vi "Teleop.vi"(10 "Match Info":T1={"Autonomous Elapsed Seconds"=0.0, "TeleOp Elapsed Seconds"=0.0, "Disabled Elapsed Seconds"=0.0, "Visited Autonomous"=FALSE, "Visited TeleOp"=FALSE, "Visited Disabled"=FALSE, "Autonomous Settings"={"Autonomous Style"=enum."Independent", "VI Refnum"=refnum}}, 11 "Call Context":T2) -> ()   [LabVIEW 2012]
doc: "This VI is called for each TeleOp packet received from the DS where the robot is not disabled. It is often used to read from the joysticks and update I/O or to update setpoints for timed control loops. It should complete and return within 20 milliseconds or it may miss DS packets."
uses:
  <vilib>/Rock Robotics/WPI/DriverStation/WPI_DriverStationDerivedRobotMode.ctl
  <vilib>/Rock Robotics/WPI/DriverStation/WPI_DriverStationMatch Info.ctl
  <vilib>/Rock Robotics/WPI/Relay/WPI_RelayValue.ctl
  Robot Global Data.vi
  <vilib>/Rock Robotics/WPI/Joystick/WPI_JoystickGetSetRefNum.vi
  <vilib>/Rock Robotics/WPI/RobotDrive/WPI_RobotDriveGetSetRefNum.vi
panel:
  out "Numeric 1":dbl(slide) scale=0.0..100.0
  out "Boolean 2":bool
  out "Boolean 1":bool
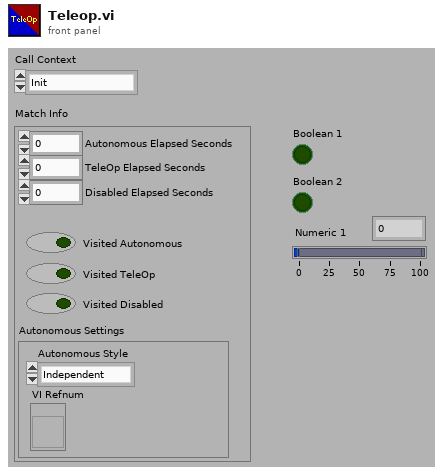
[diagram p1: front panel]
types:
  T1 = typedef "WPI_DriverStationMatch Info.ctl" = cluster{"Autonomous Elapsed Seconds":dbl, "TeleOp Elapsed Seconds":dbl, "Disabled Elapsed Seconds":dbl, "Visited Autonomous":bool, "Visited TeleOp":bool, "Visited Disabled":bool, "Autonomous Settings":cluster{"Autonomous Style":enum16{"Iterative", "Independent"}, "VI Refnum":refnum<vi>}}
  T2 = typedef "WPI_DriverStationDerivedRobotMode.ctl" = enum16{"Init", "Execute", "Stop"}
  T3 = typedef "WPI_JoystickDevRef.ctl" = cluster{"Device":T4}
  T4 = typedef "WPI_JoystickDeviceEnum.ctl" = enum16{"USB 1", "USB 2", "USB 3", "USB 4", "Kinect 1", "Kinect 2"}
  T5 = typedef "WPI_JoystickButtonState.ctl" = cluster{"Button 1":bool, "Button 2":bool, "Button 3":bool, "Button 4":bool, "Button 5":bool, "Button 6":bool, "Button 7":bool, "Button 8":bool, "Button 9":bool, "Button 10":bool, "Button 11":bool, "Button 12":bool}
  T6 = typedef "WPI_RelayValue.ctl" = enum16{"Off", "On", "Forward", "Reverse"}
  T7 = cluster{"axis 1 (x)":dbl, "axis 2 (y)":dbl, "axis 3 (throttle)":dbl, "axis 4":dbl, "axis 5":dbl, "axis 6":dbl}
  T8 = typedef "WPI_RelayDevRef.ctl" = cluster{"DevStatus":errorcluster, "Relay Channel":T9, "Digital Module":T10, "Relay Direction":T11}
  T9 = typedef "FPGA_DIORelayChannel.ctl" = enum8{"Relay 1", "Relay 2", "Relay 3", "Relay 4", "Relay 5", "Relay 6", "Relay 7", "Relay 8", "Invalid"}
  T10 = typedef "FPGA_TypedefDigitalModule.ctl" = enum16{"Digital Module 1", "Digital Module 2"}
  T11 = typedef "WPI_RelayDirection.ctl" = enum16{"Both directions", "Forward only", "Reverse only"}
  T12 = typedef "WPI_MotorControlDeviceRef.ctl" = cluster{"DeviceStatus":errorcluster, "Type":enum16{"PWM", "CAN"}, "PWM":cluster{"Digital Module":T10, "PWM Channel":T13, "DeadBand":T14}, "CAN":cluster{"Device Number":u8, "Control Mode":T15, "Semaphore":T16, "Max Vout":dbl}, "Invert":bool, "TransformRef":T17, "InvTransformRef":T17}
  T13 = typedef "FPGA_DIOPWMChannel.ctl" = enum8{"PWM 1", "PWM 2", "PWM 3", "PWM 4", "PWM 5", "PWM 6", "PWM 7", "PWM 8", "PWM 9", "PWM 10", "Invalid"}
  T14 = typedef "WPI_PWMDeadband.ctl" = cluster{"Name":string, "maxPositivePwm":i32, "minPositivePwm":i32, "centerPwm":i32, "maxNegativePwm":i32, "minNegativePwm":i32, "angularRange":u16}
  T15 = typedef "WPI_CANJaguar_ControlMode.ctl" = enum8{"Percent VBus", "Current", "Speed", "Position", "Voltage"}
  T16 = typedef "Semaphore RefNum" = refnum<k1>
  T17 = typedef "WPI_PWMTransform_ConPane.ctl" = refnum<vi>
  T18 = typedef "WPI_RobotDriveDevRef.ctl" = cluster{"DevStatus":errorcluster, "Motors[]":T12[], "Square Inputs":bool, "Max Output":dbl, "Isochronous":bool}
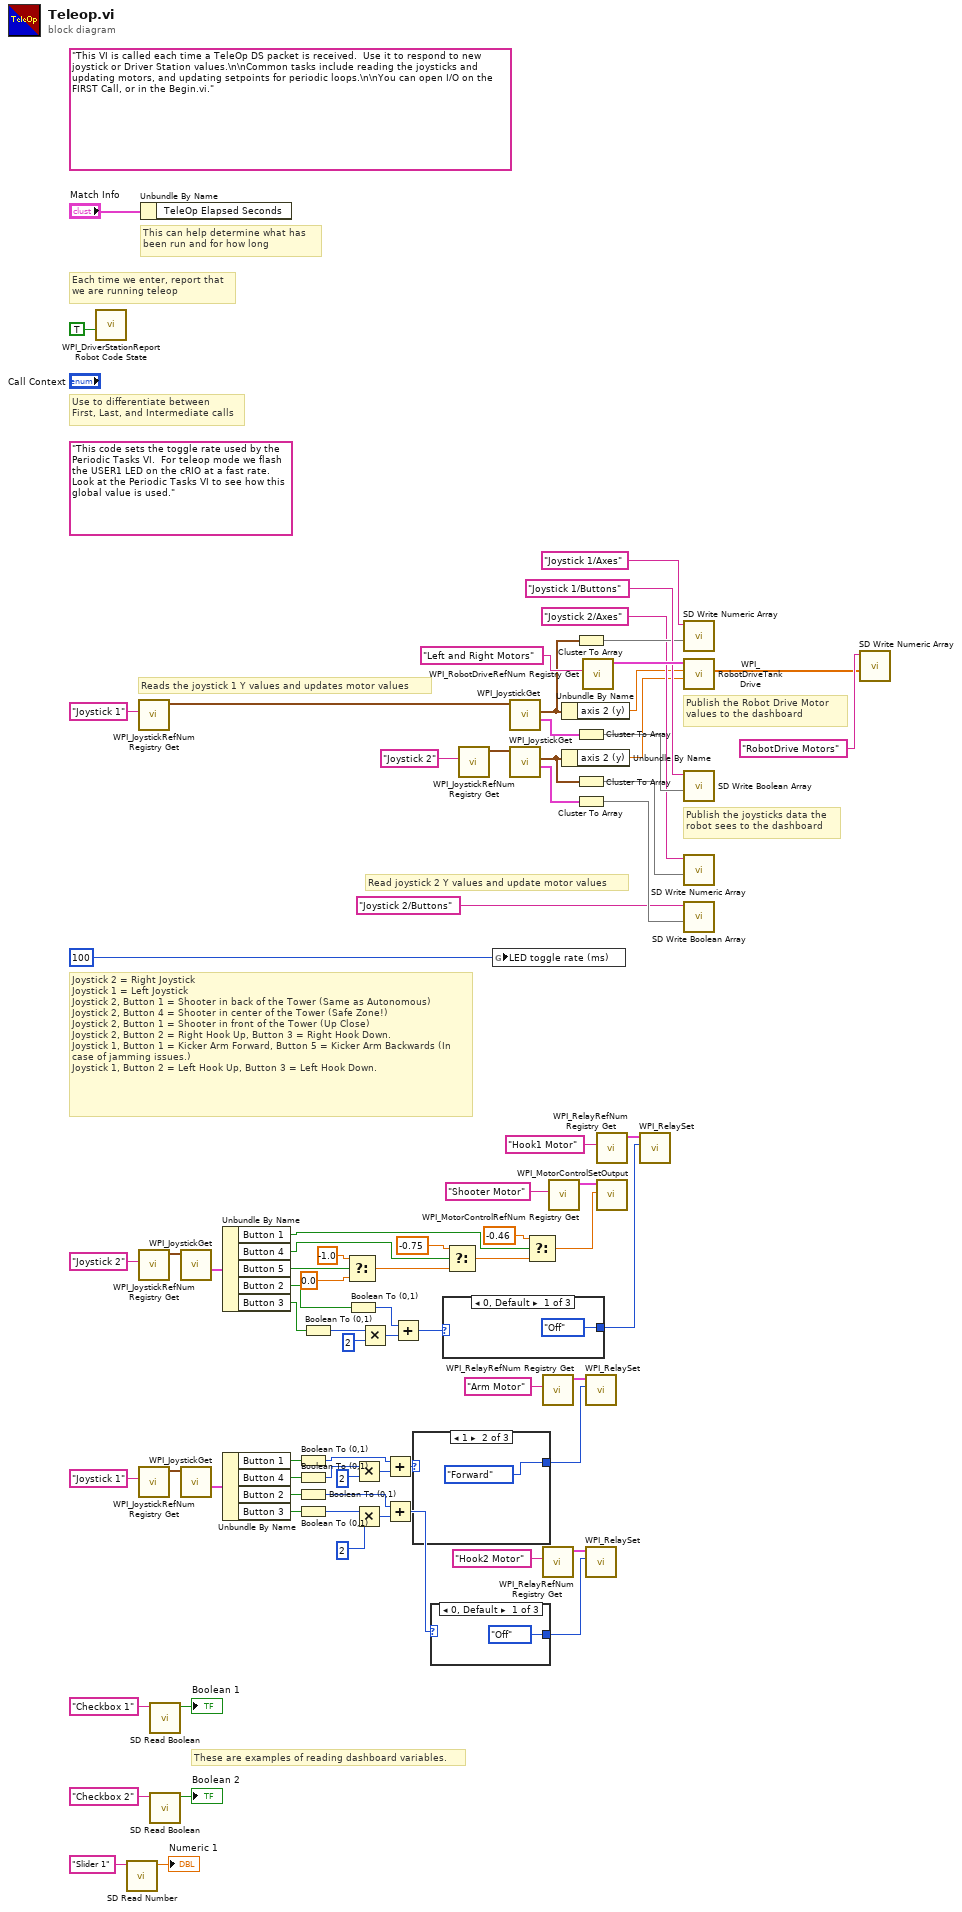
[diagram p0: block diagram]
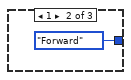
[diagram p2: hidden frame]
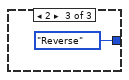
[diagram p3: hidden frame]
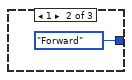
[diagram p4: hidden frame]
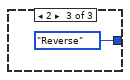
[diagram p5: hidden frame]
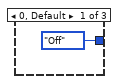
[diagram p6: hidden frame]
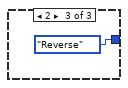
[diagram p7: hidden frame]
diagram:
  (unwired) "This code sets the toggle rate used by the Periodic Tasks VI.  For teleop mode we flash the USER1 LED on the cRIO at a fast rate.  Look at the Periodic Tasks VI to see how this global value is used."
  (unwired) "This VI is called each time a TeleOp DS packet is received.  Use it to respond to new joystick or Driver Station values.\n\nCommon tasks include reading the joysticks and updating motors, and updating setpoints for periodic loops.\n\nYou can open I/O on the FIRST Call, or in the Begin.vi."
  # "Joystick 2 = Right Joystick\nJoystick 1 = Left Joystick\nJoystick 2, Button 1 = Shooter in back of the Tower (Same as Autonomous)\nJoystick 2, Button 4 = Shooter in center of the Tower (Safe Zone!)\nJoystick 2, Button 1 = Shooter in front of the Tower (Up Close)\nJoystick 2, Button 2 = Right Hook Up, Button 3 = Right Hook Down.\nJoystick 1, Button 1 = Kicker Arm Forward, Button 5 = Kicker Arm Backwards (In case of jamming issues.)\nJoystick 1, Button 2 = Left Hook Up, Button 3 = Left Hook Down."
  # "Reads the joystick 1 Y values and updates motor values"
  # "These are examples of reading dashboard variables."
  # "Publish the Robot Drive Motor\nvalues to the dashboard"
  # "Publish the joysticks data the\nrobot sees to the dashboard"
  # "Each time we enter, report that\nwe are running teleop"
  # "Use to differentiate between\nFirst, Last, and Intermediate calls"
  # "This can help determine what has\nbeen run and for how long"
  # "Read joystick 2 Y values and update motor values"
  n1 = call <vilib>:"WPI_DriverStationReport Robot Code State.vi"("TeleOp"=TRUE ("Autonomous")) -> ()  [unwired: 10 in, 1 out]
  n2 = call <vilib>:"SD Read Number.vi"("Name"="Slider 1" ("refnum name")) -> ("Numeric"=→"Numeric 1":dbl)  [unwired: 8 in, 2 out]
  n3 = call <vilib>:"WPI_JoystickRefNum Registry Get.vi"("refnum name"="Joystick 1") -> ("JoystickDevRef"=w68:T3)  [unwired: 1 in, 9 out]
  n4 = call <vilib>:"WPI_JoystickRefNum Registry Get.vi"("refnum name"="Joystick 2") -> ("JoystickDevRef"=w47:T3)  [unwired: 1 in, 9 out]
  n5 = call <vilib>:"WPI_JoystickRefNum Registry Get.vi"("refnum name"="Joystick 1") -> ("JoystickDevRef"=w43:T3)  [unwired: 1 in, 9 out]
  n6 = Unbundle By Name("Match Info") -> ()  [unwired: 1 out]
  n7 = call <vilib>:"SD Read Boolean.vi"("Name"="Checkbox 1" ("refnum name")) -> ("Boolean"=→"Boolean 1":bool)  [unwired: 8 in, 2 out]
  n8 = call <vilib>:"SD Read Boolean.vi"("Name"="Checkbox 2" ("refnum name")) -> ("Boolean"=→"Boolean 2":bool)  [unwired: 8 in, 2 out]
  n9 = call <vilib>:"WPI_JoystickGet.vi"("JoystickDevRef"=w47) -> ("Buttons"=w46:T5)  [unwired: 1 in, 5 out]
  n10 = call <vilib>:"WPI_JoystickGet.vi"("JoystickDevRef"=w43) -> ("Buttons"=w36:T5)  [unwired: 1 in, 5 out]
  n11 = Unbundle By Name(w46) -> ("Button 1"=w29:bool, "Button 4"=w22:bool, "Button 5"=w21:bool, "Button 2"=w11:bool, "Button 3"=w12:bool)
  n12 = Unbundle By Name(w36) -> ("Button 1"=w40:bool, "Button 4"=w39:bool, "Button 2"=w2:bool, "Button 3"=w1:bool)
  n13 = Boolean To (0,1)(Boolean=w40) -> (0, 1=w38:i16)
  n14 = Boolean To (0,1)(Boolean=w39) -> (0, 1=w34:i16)
  n15 = Boolean To (0,1)(Boolean=w2) -> (0, 1=w8:i16)
  n16 = Boolean To (0,1)(Boolean=w1) -> (0, 1=w4:i16)
  n17 = Boolean To (0,1)(Boolean=w12) -> (0, 1=w14:i16)
  n18 = Select(t=-1.0, s=w21, f=0.0) -> (s? t:f=w24:dbl)
  n19 = Boolean To (0,1)(Boolean=w11) -> (0, 1=w18:i16)
  n20 = Multiply(x=w34, y=i16 2) -> (x*y=w33:i16)
  n21 = Multiply(x=w4, y=i16 2) -> (x*y=w3:i16)
  n22 = Multiply(x=w14, y=i16 2) -> (x*y=w13:i16)
  n23 = Add(x=w38, y=w33) -> (x+y=w37:i16)
  n24 = Add(x=w8, y=w3) -> (x+y=w7:i16)
  n25 = Add(x=w18, y=w13) -> (x+y=w17:i16)
  n26 = case shown="1" w37 {
    tunnel: [WPI_RelayValue."Off" ("RelayValue") WPI_RelayValue."Forward" ("RelayValue") WPI_RelayValue."Reverse" ("RelayValue")] -> w32
    frame 0, Default {
    }
    frame 1 {
    }
    frame 2 {
    }
  }
  n27 = case shown="0, Default" w7 {
    tunnel: [WPI_RelayValue."Off" ("RelayValue") WPI_RelayValue."Forward" ("RelayValue") WPI_RelayValue."Reverse" ("RelayValue")] -> w6
    frame 0, Default {
    }
    frame 1 {
    }
    frame 2 {
    }
  }
  n28 = case shown="0, Default" w17 {
    tunnel: [WPI_RelayValue."Off" ("RelayValue") WPI_RelayValue."Forward" ("RelayValue") WPI_RelayValue."Reverse" ("RelayValue")] -> w16
    frame 0, Default {
    }
    frame 1 {
    }
    frame 2 {
    }
  }
  n29 = Select(t=-0.75, s=w22, f=w24) -> (s? t:f=w23:dbl)
  n30 = call <vilib>:"WPI_JoystickRefNum Registry Get.vi"("refnum name"="Joystick 2") -> ("JoystickDevRef"=w60:T3)  [unwired: 1 in, 9 out]
  n31 = global write "Robot Global Data.vi" "LED toggle rate (ms)"(u32 100 ("LED ms toggle rate")) -> ()
  n32 = call <vilib>:"WPI_JoystickGet.vi"("JoystickDevRef"=w68) -> ("Buttons"=w67:T5, "Axes"=w62:T7)  [unwired: 1 in, 4 out]
  n33 = call <vilib>:"WPI_JoystickGet.vi"("JoystickDevRef"=w60) -> ("Buttons"=w59:T5, "Axes"=w54:T7)  [unwired: 1 in, 4 out]
  n34 = Select(t=-0.46, s=w29, f=w23) -> (s? t:f=w28:dbl)
  n35 = call <vilib>:"WPI_RelayRefNum Registry Get.vi"("refnum name"="Arm Motor") -> ("RelayDevRef"=w41:T8)  [unwired: 9 in, 1 out]
  n36 = call <vilib>:"WPI_RelayRefNum Registry Get.vi"("refnum name"="Hook2 Motor") -> ("RelayDevRef"=w9:T8)  [unwired: 9 in, 1 out]
  n37 = call <vilib>:"WPI_MotorControlRefNum Registry Get.vi"("refnum name"="Shooter Motor") -> ("MotorControlDevRef"=w31:T12)  [unwired: 9 in, 1 out]
  n38 = Unbundle By Name(w62) -> ("axis 2 (y)"=w49:dbl)
  n39 = Unbundle By Name(w54) -> ("axis 2 (y)"=w52:dbl)
  n40 = Cluster To Array(cluster=w62) -> (array=w64:dbl[])
  n41 = Cluster To Array(cluster=w67) -> (array=w66:bool[])
  n42 = Cluster To Array(cluster=w54) -> (array=w56:dbl[])
  n43 = Cluster To Array(cluster=w59) -> (array=w58:bool[])
  n44 = call <vilib>:"WPI_RobotDriveRefNum Registry Get.vi"("refnum name"="Left and Right Motors") -> ("RobotDriveDevRef"=w69:T18)  [unwired: 1 in, 9 out]
  n45 = call <vilib>:"WPI_RelaySet.vi"("RelayValue"=w32, "RelayDevRef"=w41) -> ()  [unwired: 8 in, 2 out]
  n46 = call <vilib>:"WPI_RelaySet.vi"("RelayValue"=w6, "RelayDevRef"=w9) -> ()  [unwired: 8 in, 2 out]
  n47 = call <vilib>:"WPI_RelayRefNum Registry Get.vi"("refnum name"="Hook1 Motor") -> ("RelayDevRef"=w19:T8)  [unwired: 9 in, 1 out]
  n48 = call <vilib>:"WPI_MotorControlSetOutput.vi"("Output"=w28, "MotorControlDevRef"=w31) -> ()  [unwired: 7 in, 3 out]
  n49 = call <vilib>:"WPI_RelaySet.vi"("RelayValue"=w16, "RelayDevRef"=w19) -> ()  [unwired: 8 in, 2 out]
  n50 = call <vilib>:"SD Write Numeric Array.vi"("Numeric Array"=w64, "Name"="Joystick 1/Axes") -> ()  [unwired: 8 in, 2 out]
  n51 = call <vilib>:"WPI_RobotDriveTankDrive.vi"("Right axis value"=w52, "Left axis value"=w49, "RobotDriveDevRef"=w69) -> ("Motor Values"=w50:dbl[])  [unwired: 6 in, 2 out]
  n52 = call <vilib>:"SD Write Boolean Array.vi"("Boolean Array"=w66, "Name"="Joystick 1/Buttons") -> ()  [unwired: 8 in, 2 out]
  n53 = call <vilib>:"SD Write Numeric Array.vi"("Numeric Array"=w56, "Name"="Joystick 2/Axes") -> ()  [unwired: 8 in, 2 out]
  n54 = call <vilib>:"SD Write Boolean Array.vi"("Boolean Array"=w58, "Name"="Joystick 2/Buttons") -> ()  [unwired: 8 in, 2 out]
  n55 = call <vilib>:"SD Write Numeric Array.vi"("Numeric Array"=w50, "Name"="RobotDrive Motors") -> ()  [unwired: 8 in, 2 out]
